vi "silver error cluster.vi"() -> ()   [LabVIEW 2021]
panel:
  in  "error in":errorcluster={"status"=TRUE, "code"=1, "source"="abc"}
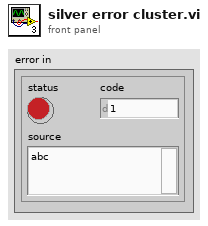
[diagram p1: front panel]
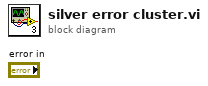
[diagram p0: block diagram]
diagram:
